vi "Serchandreplace.vi"() -> ()   [LabVIEW 2017]
panel:
  in  "stop":bool
  out "result string":string
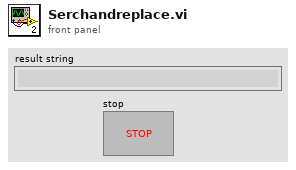
[diagram p1: front panel]
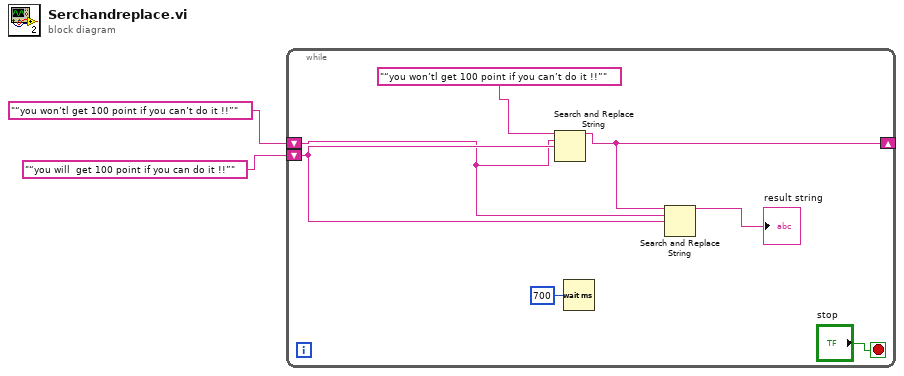
[diagram p0: block diagram]
diagram:
  n1 = while {
    shift-right: [w8] -> _
    shift-left: "“you won’tl get 100 point if you can’t do it !!”" -> [w5]
    shift-left: "“you will  get 100 point if you can do it !!”" -> [w6]
    stop <- "stop" stop-if-true
    n2 = Search and Replace String(input string="“you won’tl get 100 point if you can’t do it !!”", search string=w5, replace string=w6) -> (result string=w8:string)  [unwired: 5 in, 3 out]
    n3 = Wait (ms)(milliseconds to wait=u32 700) -> ()  [unwired: 1 out]
    n4 = Search and Replace String(input string=w8, search string=w5, replace string=w6) -> (result string=→"result string":string)  [unwired: 5 in, 3 out]
  }
